vi "Replace Object Control Labels.vi"(4 "in / out":string, 6 "Post":string, 8 "error in":errorcluster, 9 "Pre":string, 10 "VI Ref":refnum<vi>) -> (0 "error out":errorcluster)   [LabVIEW 2021, in "_Rename.lvlib" / "_Rename.lvclass"]
uses:
  _Rename.lvclass
  <vilib>/Utility/traverseref.llb/TRef TravTarget.ctl
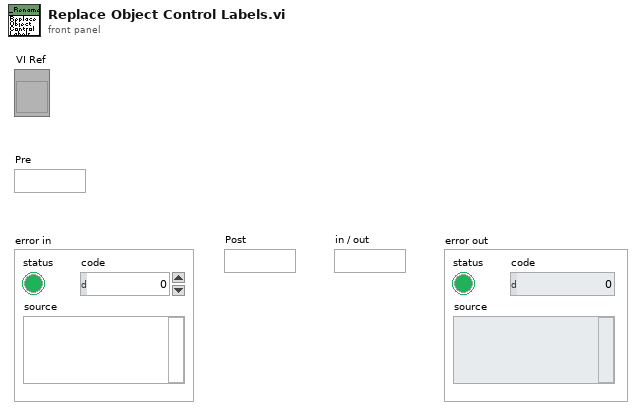
[diagram p1: front panel]
types:
  T1 = typedef "TRef TravTarget.ctl" = enum16{"FP", "BD", "Other"}
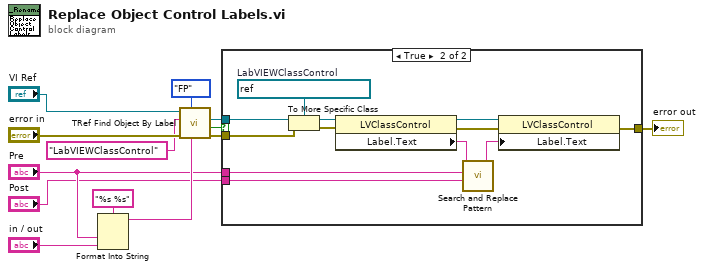
[diagram p0: block diagram]
diagram:
  n1 = Format Into String(format string="%s %s", "Pre", "in / out") -> (resulting string=w11:string)  [unwired: 2 in, 1 out]
  n2 = call <vilib>:"TRef Find Object By Label.vi"("Label"=w11, "Traverse Target"=TRef_TravTarget."FP", "error in (no error)"="error in", "Class Name"="LabVIEWClassControl", "VI Ref"="VI Ref") -> ("error out"=w10:errorcluster, "Found?"=w9:bool, "Found Obj Ref"=w13:refnum<vi>)  [unwired: 3 in, 1 out]
  n3 = case shown="True" w9 {
    tunnel: [_ w25] -> w4
    tunnel: w13 -> [_ w23]
    tunnel: w10 -> [_ w24]
    tunnel: "Pre" -> [_ w15]
    tunnel: "Post" -> [_ w14]
    frame False {
      # "The \"in\" or \"out\" doesn't exist so..\ndo nothing"
    }
    frame True {
      w22 = refnum<vi> refnum  # LabVIEWClassControl
      n4 = To More Specific Class(target class=w22, reference=w23, error in=w24) -> (specific class reference=w21:refnum<vi>, error out=w20:errorcluster)
      n5 = property class="LVClassControl"(reference=w21, error in=w20) -> (reference out=w18:refnum<vi>, error out=w19:errorcluster, "Label.Text"=w17:string)
      n6 = call <vilib>:"Search and Replace Pattern.vi"("string"=w17, "regular expression (\"\")"=w15, "replace string (\"\")"=w14) -> ("result string"=w16:string)  [unwired: 2 in, 1 out]
      n7 = property class="LVClassControl"(reference=w18, error in=w19, "Label.Text"=w16) -> (error out=w25:errorcluster)  [unwired: 1 out]
    }
  }
  "error out" <- w4
